vi "IP SETTING.vi"() -> ()   [LabVIEW 2017]
uses:
  <vilib>/addons/database/Connection.llb/DB Tools Open Connec (String).vi
  Global/Global 1.vi
  <vilib>/addons/database/NI_Database_API.lvlib
panel:
  in  "SAVE":bool
  in  "Cluster":T1
  out "error out":errorcluster
  in  "error in (no error)":errorcluster
  in  "EXIT":bool
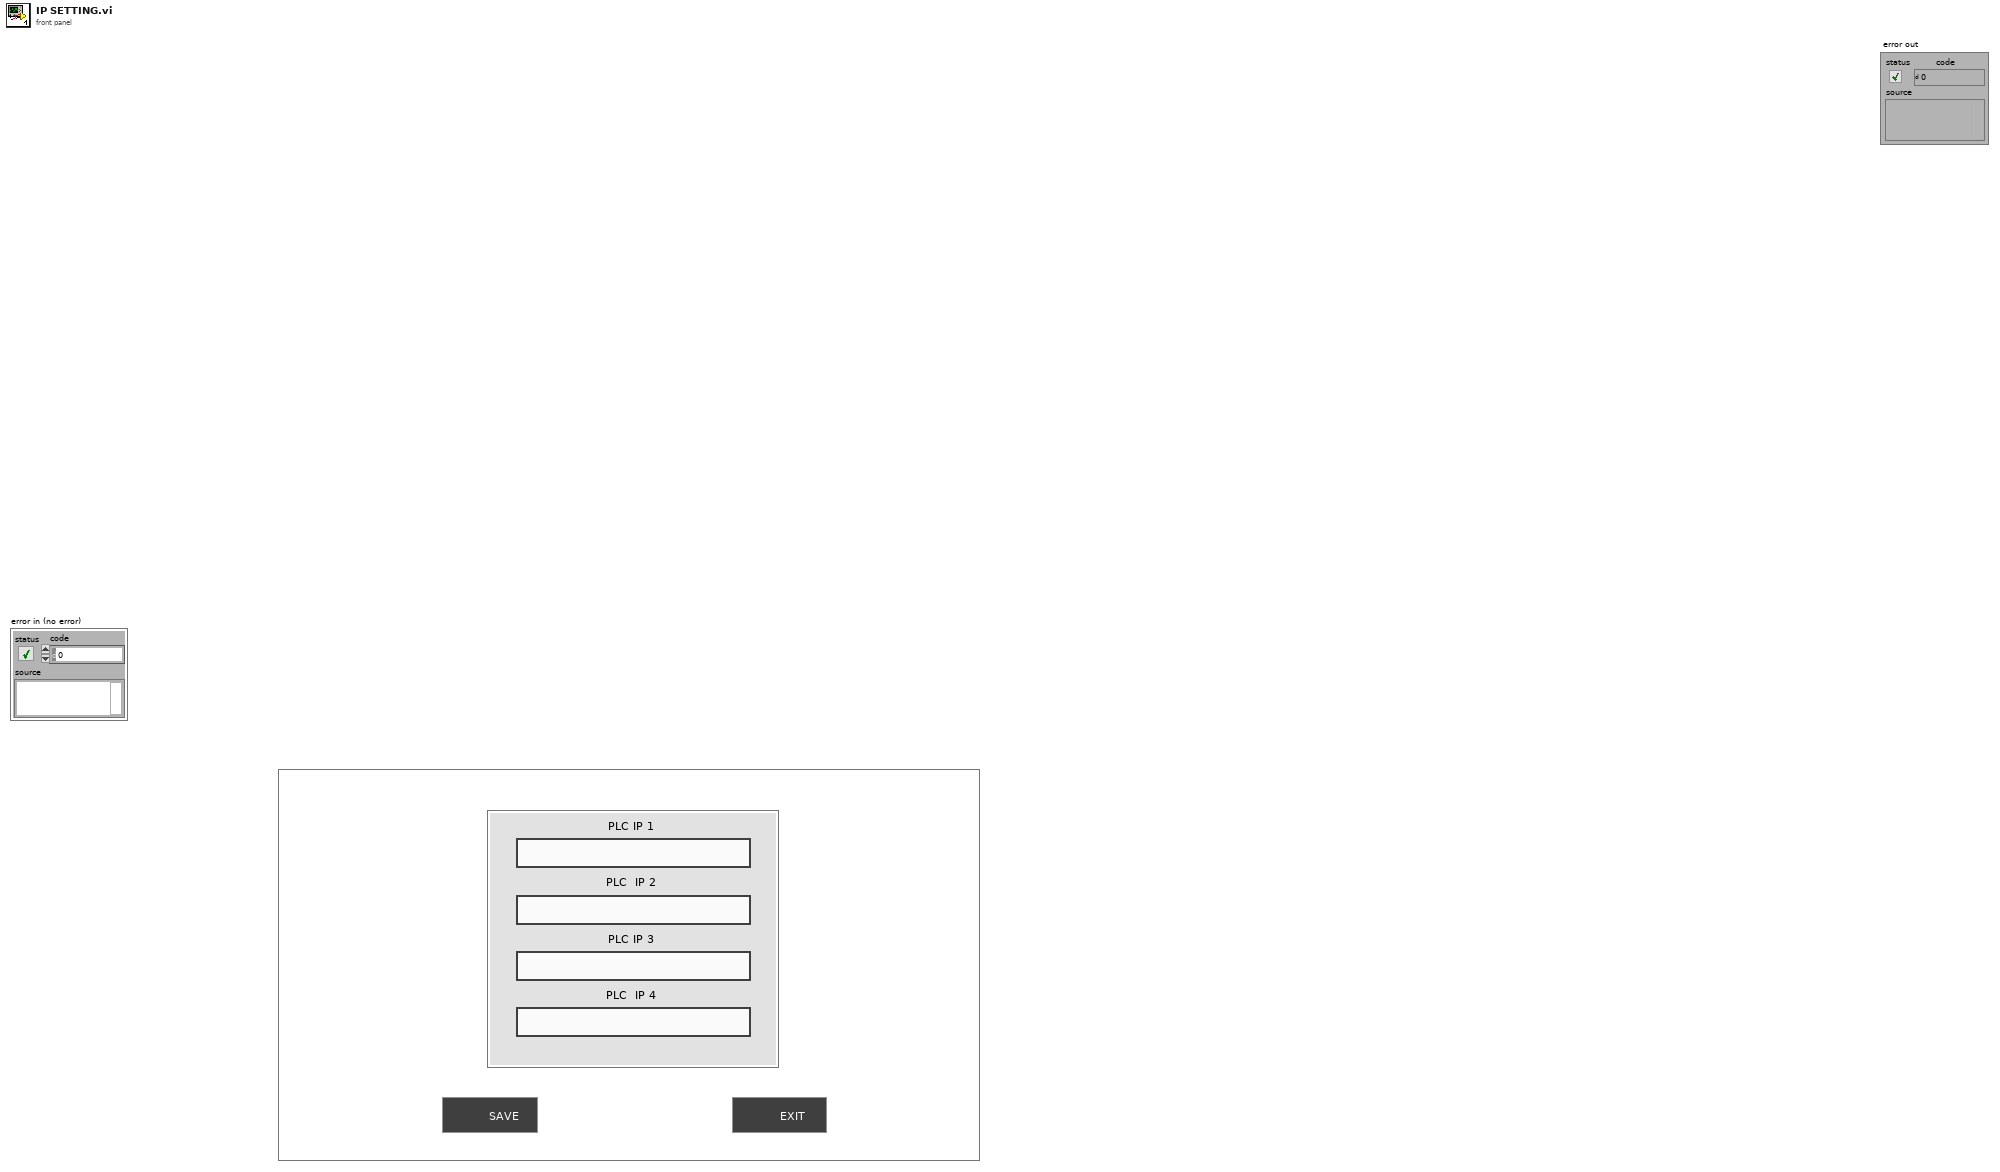
[diagram p1: front panel]
types:
  T1 = cluster{"PLC IP 1":string, "PLC  IP 2":string, "PLC IP 3":string, "PLC  IP 4":string}
  T2 = typedef "NI_Database_API.lvlib/Conn ObjectReference.ctl" = refnum<k1>
  T3 = enum32{"invalid app kind", "Development System", "Run Time System", "Student Edition", "Embedded LabVIEW", "Evaluation", "Custom"}
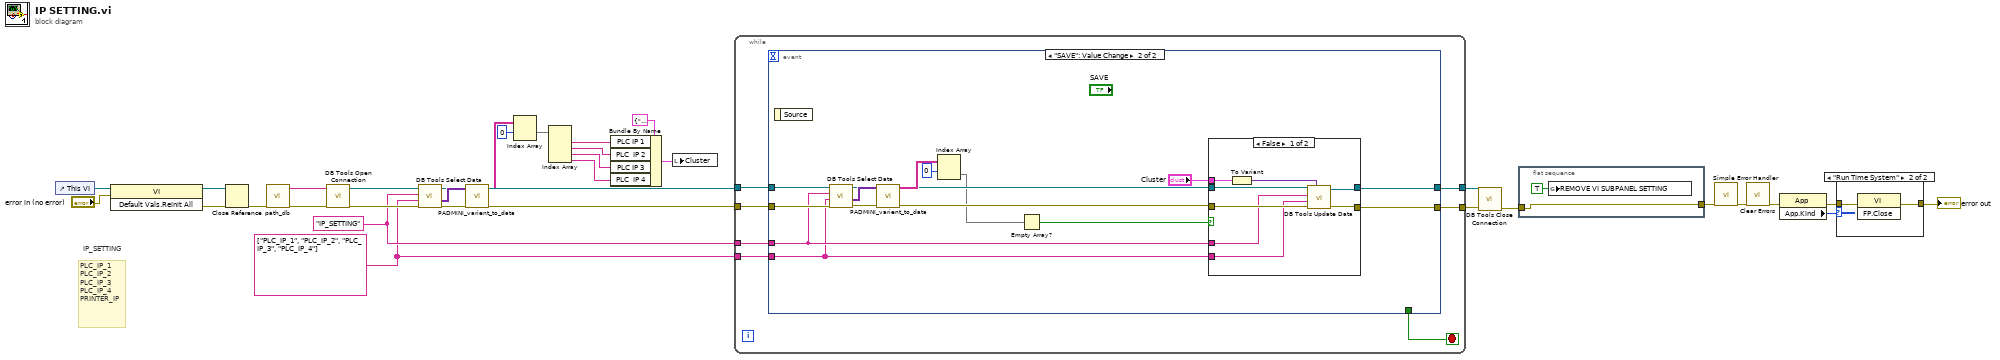
[diagram p0: block diagram]
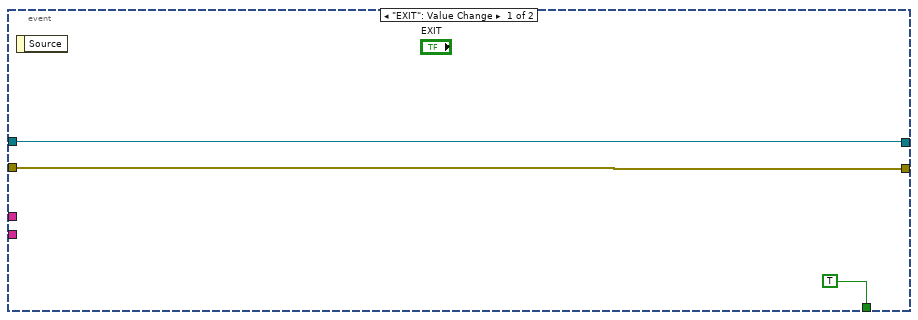
[diagram p2: hidden frame]
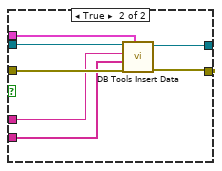
[diagram p3: hidden frame]
diagram:
  w3 = string[] ["PLC_IP_1", "PLC_IP_2", "PLC_IP_3", "PLC_IP_4"] ("columns")
  w8 = "IP_SETTING" ("table")
  # "PLC_IP_1\nPLC_IP_2\nPLC_IP_3\nPLC_IP_4\nPRINTER_IP"
  # "IP_SETTING"
  n1 = control-ref of="This VI"() -> (w33:refnum<vi>)
  n2 = invoke class="VI" method="Default Vals.Reinit All"(reference=w33, error in="error in (no error)") -> (reference out=w31:refnum<vi>, error out=w32:errorcluster)  [unwired: 1 in, 1 out]
  n3 = Close Reference(reference=w31, error in (no error)=w32) -> (error out=w23:errorcluster)
  n4 = call "path_db.vi"("error in"=w23) -> ("error out"=w16:errorcluster, "resulting string"=w21:string)  [unwired: 9 in]
  n5 = call-poly <vilib>:"DB Tools Open Connection.vi"("error in (no error)"=w16, "connection information"=w21) -> ("error out"=w20:errorcluster, "connection reference"=w19:T2)  [unwired: 6 in]
  n6 = call <vilib>:"DB Tools Select Data.vi"("error in (no error)"=w20, "columns"=w3, "table"=w8, "connection reference"=w19) -> ("error out"=w18:errorcluster, "data"=w17:variant[][], "connection reference out"=w11:T2)  [unwired: 2 in]
  n7 = call "PADMINI_varient_to_data.vi"("error in (no error)"=w18, "data"=w17) -> ("error out"=w15:errorcluster, "Array"=w10:string[][])  [unwired: 8 in]
  n8 = Index Array(array=w10, index (row)=0 ("disabled index (col)")) -> (element=w9:string[])  [unwired: 1 in]
  n9 = Index Array(array=w9) -> (element #1=w14:string, element #2=w13:string, element #3=w12:string, element #4=w1:string)  [unwired: 4 in]
  n10 = Bundle By Name(cluster=T1 {"PLC IP 1"="", "PLC  IP 2"="", "PLC IP 3"="", "PLC  IP 4"=""} ("Cluster"), "PLC IP 1"=w14, "PLC  IP 2"=w13, "PLC IP 3"=w12, "PLC  IP 4"=w1) -> (w22:T1)
  n11 = local write "Cluster"(w22) -> ()
  n12 = while {
    tunnel: [w39] -> w6
    tunnel: w15 -> [w40]
    tunnel: w11 -> [w37]
    tunnel: [w36] -> w7
    tunnel: w8 -> [w35]
    tunnel: w3 -> [w34]
    stop <- w38 stop-if-true
    n13 = event shown="[1] \"SAVE\": Value Change" {
      selector: _ -> [_ _]
      dyn-events: _ -> [_ _]
      timeout: _ -> [_ _]
      tunnel: w40 -> [w43 w50]
      tunnel: [w43 w58] -> w39
      tunnel: [TRUE _] -> w38
      tunnel: w37 -> [w41 w51]
      tunnel: [w41 w57] -> w36
      tunnel: w35 -> [_ w49]
      tunnel: w34 -> [_ w48]
      event "EXIT": Value Change {
        n14 = event-data() -> ()  [unwired: 1 in, 1 out]
      }
      event "SAVE": Value Change {
        n15 = event-data() -> ()  [unwired: 1 in, 1 out]
        n16 = call <vilib>:"DB Tools Select Data.vi"("error in (no error)"=w50, "columns"=w48, "table"=w49, "connection reference"=w51) -> ("error out"=w52:errorcluster, "data"=w53:variant[][], "connection reference out"=w46:T2)  [unwired: 2 in]
        n17 = call "PADMINI_varient_to_data.vi"("error in (no error)"=w52, "data"=w53) -> ("error out"=w47:errorcluster, "Array"=w54:string[][])  [unwired: 8 in]
        n18 = Index Array(array=w54, index (row)=0 ("disabled index (col)")) -> (element=w45:string[])  [unwired: 1 in]
        n19 = Empty Array?(array=w45) -> (empty?=w44:bool)
        n20 = case shown="False" w44 {
          tunnel: w47 -> [w65 w73]
          tunnel: w46 -> [w66 w71]
          tunnel: [w63 w72] -> w58
          tunnel: [w64 w70] -> w57
          tunnel: w49 -> [w62 w69]
          tunnel: w48 -> [w61 w68]
          tunnel: "Cluster" -> [w60 w67]
          frame False {
            n21 = To Variant(anything=w60) -> (Variant=w59:variant)
            n22 = call <vilib>:"DB Tools Update Data.vi"("data"=w59, "error in (no error)"=w65, "columns"=w61, "table"=w62, "connection reference"=w66) -> ("error out"=w63:errorcluster, "connection reference out"=w64:T2)  [unwired: 5 in]
          }
          frame True {
            n23 = call <vilib>:"DB Tools Insert Data.vi"("data"=w67, "error in (no error)"=w73, "columns"=w68, "table"=w69, "connection reference"=w71) -> ("error out"=w72:errorcluster, "connection reference out"=w70:T2)  [unwired: 5 in]
          }
        }
      }
    }
  }
  n24 = call <vilib>:"DB Tools Close Connection.vi"("error in (no error)"=w6, "connection reference"=w7) -> ("error out"=w5:errorcluster)  [unwired: 5 in]
  n25 = flat-sequence {
    tunnel: w5 -> [w75]
    tunnel: [w75] -> w24
    frame #0 {
      n26 = global write "Global 1.vi" "REMOVE VI SUBPANEL SETTING"(TRUE ("REMOVE_VI _SUBPANEL_3")) -> ()
    }
  }
  n27 = call <vilib>:"Simple Error Handler.vi"("error in (no error)"=w24) -> ("error out"=w29:errorcluster)  [unwired: 4 in, 4 out]
  n28 = call <vilib>:"Clear Errors.vi"("error in (no error)"=w29) -> ("error out"=w26:errorcluster)  [unwired: 5 in, 1 out]
  n29 = property class="App"(error in=w26) -> (error out=w27:errorcluster, "App.Kind"=w28:T3)  [unwired: 1 in, 1 out]
  n30 = case shown="\"Run Time System\"" w28 {
    tunnel: w27 -> [w76 w78]
    tunnel: [w76 w77] -> w25
    frame Default {
    }
    frame "Run Time System" {
      n31 = invoke class="VI" method="FP.Close"(error in=w78) -> (error out=w77:errorcluster)  [unwired: 2 in, 2 out]
    }
  }
  "error out" <- w25
